vi "CopyImageMaskGreyscale.vi"(8 "error in (no error)":errorcluster, 9 "Greyscale Image Mask":refnum<data-value>, 10 "Greyscale Image Destination":refnum<data-value>, 11 "Greyscale Image Source":refnum<data-value>) -> (0 "error out":errorcluster, 3 "Greyscale Image Destination (duplicate)":refnum<data-value>)   [LabVIEW 2020, in "g_ar_toolkit.image.lvlib"]
uses:
  g_ar_toolkit.image.lvlib
  g_ar_toolkit.common/Module Path.vi
  <vilib>/Utility/error.llb/Error Cluster From Error Code.vi
  1519c485-f8d8-4564-b4f6-4c035770646f.vi
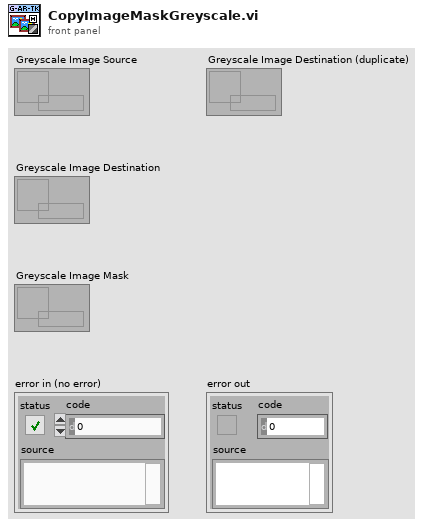
[diagram p1: front panel]
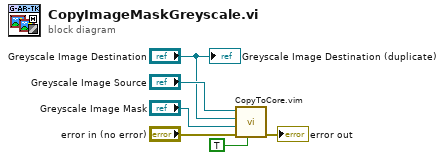
[diagram p0: block diagram]
diagram:
  n1 = call "CopyToCore.vim"("Has Mask"=TRUE, "error in (no error)"="error in (no error)", "Mask"="Greyscale Image Mask", "Dst"="Greyscale Image Destination", "Src"="Greyscale Image Source") -> ("error out"=→"error out":errorcluster)  [unwired: 6 in]
  "Greyscale Image Destination (duplicate)" <- "Greyscale Image Destination"
